vi "Rotation_GetRotations.vi"(11 "in ROTATION":T1={"VALUE"=0.0, "COS"=1.0, "SIN"=0.0} {"SIN" format="%13.4f"; "COS" format="%13.4f"; "VALUE" format="%13.4f"}) -> (3 "AngleRotations":dbl)   [LabVIEW 2019, in "Trajectory_Library.lvlib"]
doc: "Get the angle in degrees from the rotation.\n\nParameters:\n- ROTATION - The rotation data structure\n\nResults:\n- Angle in rotations."
uses:
  ROTATION2D.ctl
  Trajectory_Library.lvlib
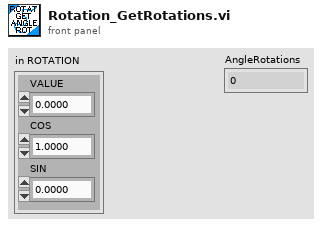
[diagram p1: front panel]
types:
  T1 = typedef "Trajectory_Library.lvlib/ROTATION2D.ctl" = cluster{"VALUE":dbl, "COS":dbl, "SIN":dbl}
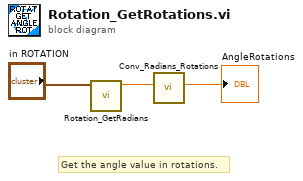
[diagram p0: block diagram]
diagram:
  # "Get the angle value in rotations."
  n1 = call "Rotation_GetRadians.vi"("in ROTATION"="in ROTATION") -> ("AngleRadians"=w2:dbl)  [unwired: 10 in]
  n2 = call "Conv_Radians_Rotations.vi"("Radians"=w2) -> ("Rotations"=→"AngleRotations":dbl)  [unwired: 10 in]
